vi ".dat File Creator for RatTracker.vi"(11 "Path of Folder with .avi and .dat":path) -> (3 "Reference to .dat File":refnum<file>)   [LabVIEW 2014]
doc: "Takes in location of folder for recording session. Creates a .dat file with the appropraite column headers and outputs a reference to this .dat file."
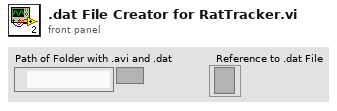
[diagram p1: front panel]
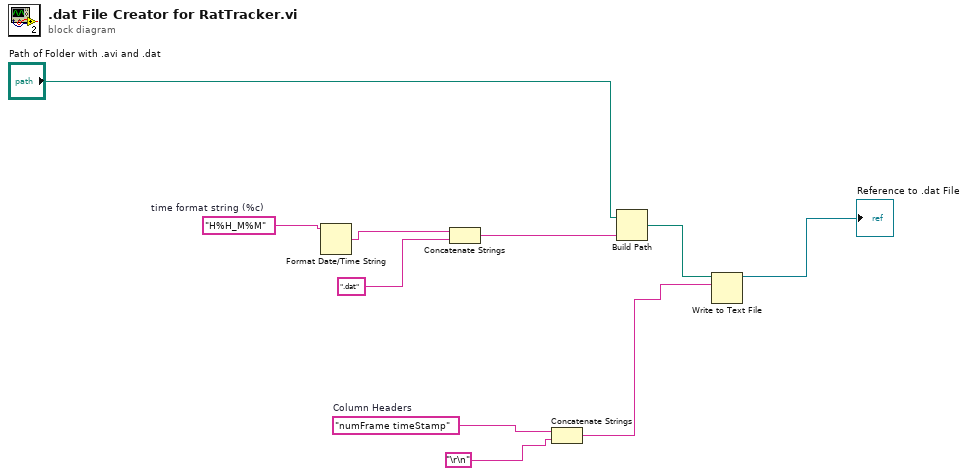
[diagram p0: block diagram]
diagram:
  w5 = "H%H_M%M"  # time format string (%c)
  w3 = "numFrame timeStamp"  # Column Headers
  n1 = Format Date/Time String(time format string (%c)=w5) -> (date/time string=w6:string)  [unwired: 2 in]
  n2 = Concatenate Strings(w6, ".dat") -> (w8:string)
  n3 = Concatenate Strings(w3, "\r\n") -> (w4:string)
  n4 = Build Path(base path="Path of Folder with .avi and .dat", name or relative path=w8) -> (appended path=w10:path)
  n5 = Write to Text File(file (use dialog)=w10, text=w4) -> (refnum out=→"Reference to .dat File":refnum<file>)  [unwired: 2 in, 2 out]
